vi "SLL DE DI Engine.vi"(8 "error in (no error)":errorcluster, 11 "Delay (ms)":u32=100) -> (0 "error out":errorcluster)   [LabVIEW 2013]
doc: "Copyright © 2005, Soliton Technologies.\nAll rights reserved."
uses:
  Controls/SLL DE DAQ Engine Options.ctl
  Controls/SLL DE DAQ Engine Channel Types.ctl
  Controls/SLL DE DAQ Global Options.ctl
  Controls/SLL DE DAQ Global Elements.ctl
  Controls/SLL DE DI Global Options.ctl
  <vilib>/DAQmx/read.llb/DAQmx Read (Digital 1D Bool NChan 1Samp 1Line).vi
  <vilib>/DAQmx/miscellaneous.llb/DAQmx Fill In Error Info.vi
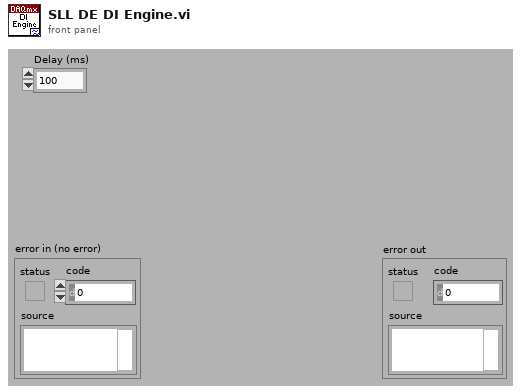
[diagram p1: front panel]
types:
  T1 = typedef "SLL DE DAQ Engine Options.ctl" = enum16{">Init", ">Safe Mode", ">Poll", ">Error", ">Exit", ">Restart", ">DI", ">DO", ">AI", ">AO", ">Start Task", ">Stop Task"}
  T2 = typedef "SLL DE DAQ Global Options.ctl" = enum16{"Init", "Write 1", "Read 1", "Write Array", "Read Array", "Clear"}
  T3 = typedef "SLL DE DAQ Engine Channel Types.ctl" = enum16{"Analog Input", "Analog Output", "Digital Input", "Digital Output"}
  T4 = cluster{"DI Data":bool[], "Array of Tasks":refnum<k21>[], "Channel Order":i32[]}
  T5 = typedef "SLL DE DI Global Options.ctl" = enum16{"Init", "Write Line", "Write Array", "Read Line", "Read Array", "Read Full Status", "Write Full Status"}
  T6 = typedef "SLL DE DAQ Global Elements.ctl" = enum16{"AI Error", "AO Error", "DI Error", "DO Error", "AI Restart", "DI Restart", "AI Running", "AO Running", "DI Running", "DO Running", "DAQ Exit?"}
  T7 = enum16{"Left Button", "Center Button", "Right Button", "Window Close"}
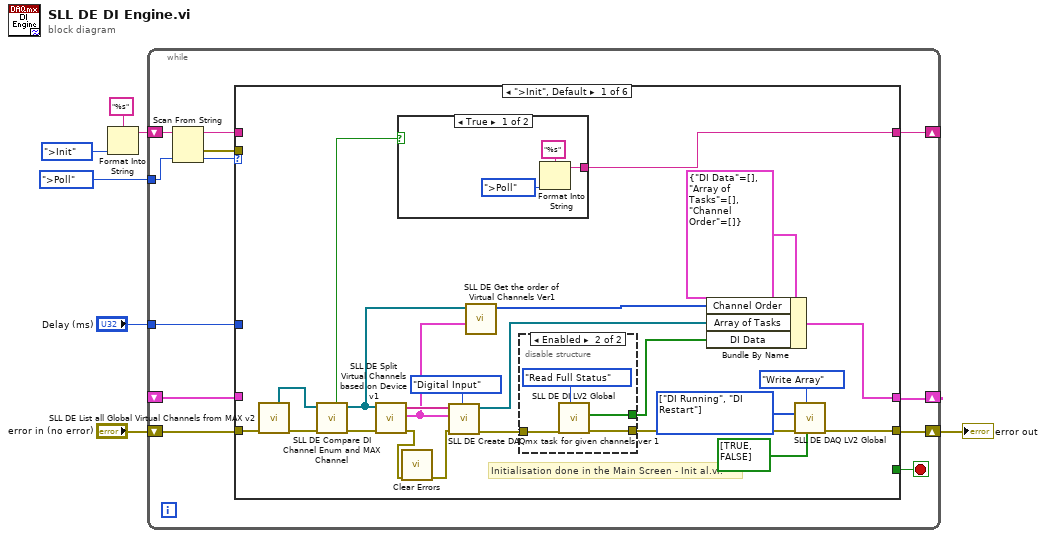
[diagram p0: block diagram]
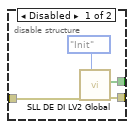
[diagram p2: hidden frame]
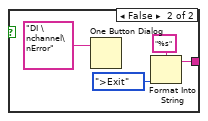
[diagram p3: hidden frame]
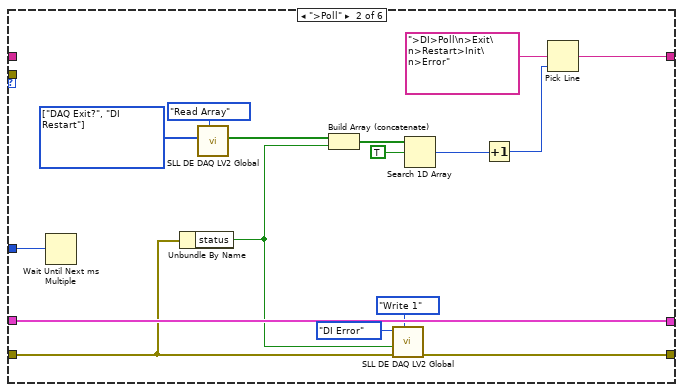
[diagram p4: hidden frame]
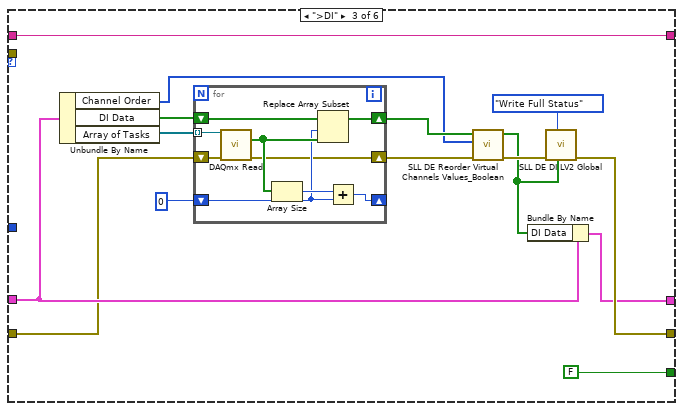
[diagram p5: hidden frame]
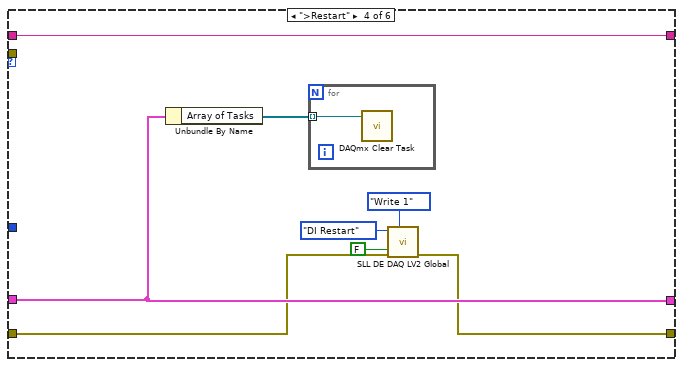
[diagram p6: hidden frame]
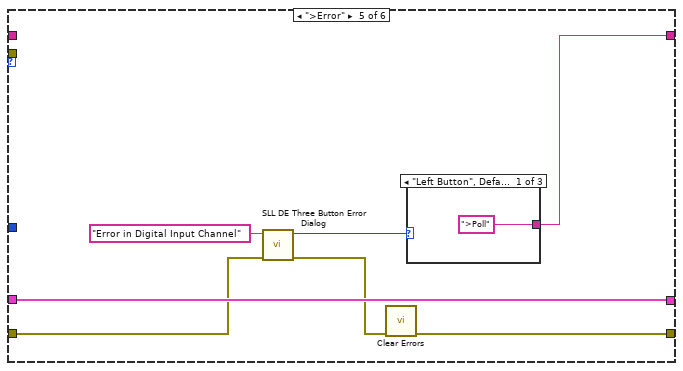
[diagram p7: hidden frame]
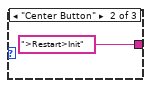
[diagram p8: hidden frame]
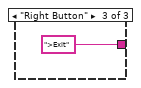
[diagram p9: hidden frame]
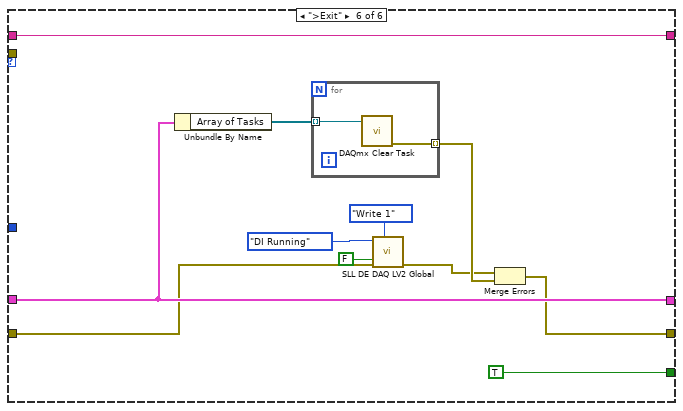
[diagram p10: hidden frame]
diagram:
  n1 = Format Into String(format string="%s", SLL_DE_DAQ_Engine_Options.">Init" ("DAQ Options")) -> (resulting string=w3:string)  [unwired: 2 in, 1 out]
  n2 = while {
    shift-right: [w18] -> w6
    shift-left: "error in (no error)" -> [w19]
    shift-right: [w17] -> _
    shift-left: _ -> [w16]
    shift-right: [w12] -> _
    shift-left: w3 -> [w15]
    tunnel: "Delay (ms)" -> [w10]
    tunnel: SLL_DE_DAQ_Engine_Options.">Poll" ("DAQ Options") -> [w8]
    stop <- w11 stop-if-true
    n3 = Scan From String(input string=w15, default 1=w8) -> (remaining string=w14:string, error out=w13:errorcluster, output 1=w9:T1)  [unwired: 3 in, 1 out]
    n4 = case shown="\">Init\", Default" w9 {
      tunnel: w19 -> [w39 w63 w75 w99 w111 w117]
      tunnel: [w35 w62 w86 w98 w109 w122] -> w18
      tunnel: [w41 w73 w77 w104 w113 w125] -> w17
      tunnel: w16 -> [_ w73 w78 w104 w113 w125]
      tunnel: w14 -> [_ _ w88 w105 _ w127]
      tunnel: w13 -> [_ _ _ _ _ _]
      tunnel: [w38 w67 w88 w105 w107 w127] -> w12
      tunnel: [_ _ FALSE _ _ TRUE] -> w11
      tunnel: w10 -> [_ w66 _ _ _ _]
      frame ">Init", Default {
        w34 = T6[] [enum."DI Running", enum."DI Restart"] items=["AI Error", "AO Error", "DI Error", "DO Error", "AI Restart", "DI Restart", "AI Running", "AO Running", "DI Running", "DO Running", "DAQ Exit?"] ("Elements Array")
        # "Initialisation done in the Main Screen - Init al.vi."
        n5 = call "SLL DE List all Global Virtual Channels from MAX v2.vi"("error in (no error)"=w39) -> ("error out"=w23:errorcluster, "Digital Input"=w26:refnum<k21>[])  [unwired: 4 in, 5 out]
        n6 = call "SLL DE Compare DI Channel Enum and MAX Channel.vi"("error in (no error)"=w23, "Digital Input Channels"=w26) -> ("error out"=w22:errorcluster, "Channels Out"=w24:refnum<k21>[], "Pass?"=w25:bool)  [unwired: 7 in]
        n7 = call "SLL DE Split Virtual Channels based on Device v1.vi"("error in (no error)"=w22, "GlobalChans"=w24) -> ("error out"=w21:errorcluster, "Channel Array"=w28:cluster{"Device Channel List":string[]}[], "Devices Names"=w32:string[])  [unwired: 7 in]
        n8 = case shown="True" w25 {
          tunnel: [w51 w55] -> w38
          frame True {
            n9 = Format Into String(format string="%s", SLL_DE_DAQ_Engine_Options.">Poll" ("DAQ Options")) -> (resulting string=w51:string)  [unwired: 2 in, 1 out]
          }
          frame False {
            n10 = One Button Dialog(message="DI \nchannel\nError") -> ()  [unwired: 1 in, 1 out]
            n11 = Format Into String(format string="%s", SLL_DE_DAQ_Engine_Options.">Exit" ("DAQ Options")) -> (resulting string=w55:string)  [unwired: 2 in, 1 out]
          }
        }
        n12 = call <vilib>:"Clear Errors.vi"("error in (no error)"=w21) -> ("error out"=w20:errorcluster)  [unwired: 6 in]
        n13 = call "SLL DE Create DAQmx task for given channels ver 1.vi"("Channel Type"=SLL_DE_DAQ_Engine_Channel_Types."Digital Input", "error in (no error)"=w20, "Channel Array"=w28, "Devices Names"=w32) -> ("error out"=w29:errorcluster, "Array of Tasks"=w30:refnum<k21>[])  [unwired: 6 in]
        n14 = call "SLL DE Get the order of Virtual Channels Ver1.vi"("Channel Array"=w28, "Virtial Channels Info"=w24) -> ("Channel Order"=w27:i32[])  [unwired: 8 in, 1 out]
        n15 = disable-structure shown="Enabled" {
          disable-tunnel: [w45 w49] -> w40
          disable-tunnel: [w44 w48] -> w36
          disable-tunnel: w29 -> [w43 w47]
          frame Disabled {
            n16 = call "SLL DE DI LV2 Global.vi"("Option"=SLL_DE_DI_Global_Options."Init", "error in (no error)"=w43) -> ("error out"=w44:errorcluster, "Digital Array Status"=w45:bool[])  [unwired: 6 in, 2 out]
          }
          frame Enabled {
            n17 = call "SLL DE DI LV2 Global.vi"("Option"=SLL_DE_DI_Global_Options."Read Full Status", "error in (no error)"=w47) -> ("error out"=w48:errorcluster, "Digital Array Status"=w49:bool[])  [unwired: 6 in, 2 out]
          }
        }
        n18 = Bundle By Name(cluster=T4 {"DI Data"=[], "Array of Tasks"=[], "Channel Order"=[]} ("Data Cluster"), "Channel Order"=w27, "Array of Tasks"=w30, "DI Data"=w40) -> (w41:T4)
        n19 = call "SLL DE DAQ LV2 Global.vi"("Status Array In"=bool[] [TRUE, FALSE], "Option"=SLL_DE_DAQ_Global_Options."Write Array", "error in (no error)"=w36, "Elements Array"=w34) -> ("error out"=w35:errorcluster)  [unwired: 5 in, 2 out]
      }
      frame ">Poll" {
        w59 = T6[] [enum."DAQ Exit?", enum."DI Restart"] items=["AI Error", "AO Error", "DI Error", "DO Error", "AI Restart", "DI Restart", "AI Running", "AO Running", "DI Running", "DO Running", "DAQ Exit?"] ("Elements Array")
        n20 = Wait Until Next ms Multiple(millisecond multiple=w66) -> ()  [unwired: 1 out]
        n21 = Unbundle By Name(w63) -> ("status"=w61:bool)
        n22 = call "SLL DE DAQ LV2 Global.vi"("Option"=SLL_DE_DAQ_Global_Options."Read Array", "Elements Array"=w59) -> ("Status Array Out"=w58:bool[])  [unwired: 7 in, 2 out]
        n23 = Build Array (concatenate)(w58, w61) -> (w71:bool[])
        n24 = call "SLL DE DAQ LV2 Global.vi"("Option"=SLL_DE_DAQ_Global_Options."Write 1", "error in (no error)"=w63, "Status In"=w61, "Element"=SLL_DE_DAQ_Global_Elements."DI Error") -> ("error out"=w62:errorcluster)  [unwired: 5 in, 2 out]
        n25 = Search 1D Array(1D array=w71, element=TRUE) -> (index of element=w69:i32)  [unwired: 1 in]
        n26 = Increment(x=w69) -> (x+1=w68:i32)
        n27 = Pick Line(multi-line string=">DI>Poll\n>Exit\n>Restart>Init\n>Error", line index=w68) -> (output string=w67:string)  [unwired: 1 in]
      }
      frame ">DI" {
        n28 = Unbundle By Name(w78) -> ("Channel Order"=w80:i32[], "DI Data"=w83:bool[], "Array of Tasks"=w84:refnum<k21>[])
        n29 = for {
          tunnel: w84 -> [w97] mode=indexing
          shift-right: [w95] -> w81
          shift-left: w83 -> [w96]
          shift-right: [w91] -> _
          shift-left: 0 -> [w92]
          shift-right: [w89] -> w74
          shift-left: w75 -> [w90]
          n30 = call-poly <vilib>:"DAQmx Read.vi"("task/channels in"=w97, "error in"=w90) -> ("data"=w94:bool[], "error out"=w89:errorcluster)  [unwired: 11 in, 1 out]
          n31 = Array Size(array=w94) -> (size(s)=w93:i32)
          n32 = Replace Array Subset(array=w96, new element=w94, index=w92) -> (w95:bool[])
          n33 = Add(x=w93, y=w92) -> (x+y=w91:i32)
        }
        n34 = call "SLL DE Reorder Virtual Channels Values_Boolean.vi"("error in (no error)"=w74, "Channel Order"=w80, "Disordered DI Data"=w81) -> ("error out"=w79:errorcluster, "Ordered DI Data"=w76:bool[])  [unwired: 7 in]
        n35 = Bundle By Name(cluster=w78, "DI Data"=w76) -> (w77:T4)
        n36 = call "SLL DE DI LV2 Global.vi"("DI State Array"=w76, "Option"=SLL_DE_DI_Global_Options."Write Full Status", "error in (no error)"=w79) -> ("error out"=w86:errorcluster)  [unwired: 5 in, 3 out]
      }
      frame ">Restart" {
        n37 = Unbundle By Name(w104) -> ("Array of Tasks"=w103:refnum<k21>[])
        n38 = for {
          tunnel: w103 -> [w106] mode=indexing
          n39 = call <vilib>:"DAQmx Clear Task.vi"("task in"=w106) -> ()  [unwired: 14 in, 1 out]
        }
        n40 = call "SLL DE DAQ LV2 Global.vi"("Option"=SLL_DE_DAQ_Global_Options."Write 1", "error in (no error)"=w99, "Status In"=FALSE, "Element"=SLL_DE_DAQ_Global_Elements."DI Restart") -> ("error out"=w98:errorcluster)  [unwired: 5 in, 2 out]
      }
      frame ">Error" {
        n41 = call "SLL DE Three Button Error Dialog.vi"("Error In"=w111, "Window Title"="Error in Digital Input Channel") -> ("Error Out"=w110:errorcluster, "Which Button?"=w108:T7)  [unwired: 8 in]
        n42 = call <vilib>:"Clear Errors.vi"("error in (no error)"=w110) -> ("error out"=w109:errorcluster)  [unwired: 6 in]
        n43 = case shown="\"Left Button\", Default" w108 {
          tunnel: [">Poll" ("Window Title") ">Restart>Init" ("Window Title") ">Exit" ("Window Title")] -> w107
          frame "Left Button", Default {
          }
          frame "Center Button" {
          }
          frame "Right Button" {
          }
        }
      }
      frame ">Exit" {
        n44 = Unbundle By Name(w125) -> ("Array of Tasks"=w124:refnum<k21>[])
        n45 = for {
          tunnel: w124 -> [w129] mode=indexing
          tunnel: [w128] -> w123 mode=indexing
          n46 = call <vilib>:"DAQmx Clear Task.vi"("task in"=w129) -> ("error out"=w128:errorcluster)  [unwired: 14 in]
        }
        n47 = call "SLL DE DAQ LV2 Global.vi"("Option"=SLL_DE_DAQ_Global_Options."Write 1", "error in (no error)"=w117, "Status In"=FALSE, "Element"=SLL_DE_DAQ_Global_Elements."DI Running") -> ("error out"=w118:errorcluster)  [unwired: 5 in, 2 out]
        n48 = Merge Errors(w118, w123) -> (w122:errorcluster)
      }
    }
  }
  "error out" <- w6
